vi "niRFUtil MEAS Peak Phase Correlation.vi"(2 "Pattern Signal":T1 {"y" format="%.2f"; "dx" format="%^.2e"; "x0" format="%^.2e"}, 3 "Signal In":T1 {"y" format="%.2f"; "dx" format="%^.2e"; "x0" format="%^.2e"}) -> (0 "Offset (s)":dbl format="%^.2e", 1 "Correlation Peak":sgl format="%^.2e")   [LabVIEW 2015, in "niRFUtil.lvlib"]
doc: "(c) Copyright 2006, National Instruments, Inc. This VI may not be duplicated, sold, or distributed without written consent from National Instruments."
uses:
  niRFUtil.lvlib
  Includes/niRFUtil INC Complex Waveform.ctl
  Includes/niRFUtil INC Complex Array.ctl
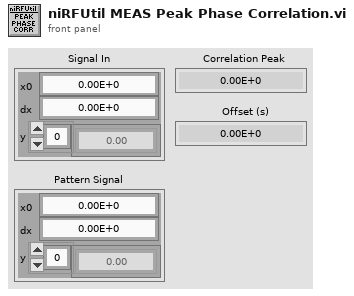
[diagram p1: front panel]
types:
  T1 = typedef "niRFUtil.lvlib/niRFUtil INC Complex Waveform.ctl" = cluster{"x0":dbl, "dx":dbl, "y":T2}
  T2 = typedef "niRFUtil.lvlib/niRFUtil INC Complex Array.ctl" = csg[]
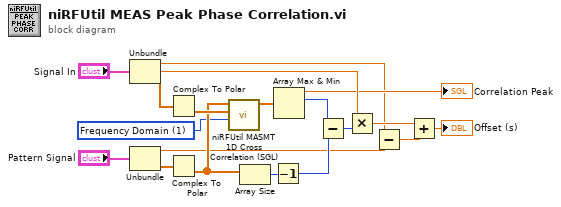
[diagram p0: block diagram]
diagram:
  w1 = 1 items=["Direct", "Frequency Domain"] ("algorithm")
  n1 = Unbundle("Signal In") -> ("x0"=w6:dbl, "dx"=w17:dbl, "y"=w3:T2)
  n2 = Unbundle("Pattern Signal") -> ("x0"=w5:dbl, "y"=w11:T2)  [unwired: 1 out]
  n3 = Complex To Polar(r * e^(i*theta)=w3) -> (theta=w19:sgl[])  [unwired: 1 out]
  n4 = Complex To Polar(r * e^(i*theta)=w11) -> (theta=w14:sgl[])  [unwired: 1 out]
  n5 = call "niRFUtil MASMT 1D Cross Correlation (SGL).vi"("algorithm"=w1, "Y"=w19, "X"=w14) -> ("Rxy"=w18:sgl[])  [unwired: 7 in, 1 out]
  n6 = Array Size(array=w14) -> (size(s)=w13:i32)
  n7 = Decrement(x=w13) -> (x-1=w12:i32)
  n8 = Array Max & Min(array=w18) -> (max value=→"Correlation Peak":sgl, max index (indices)=w16:i32)  [unwired: 2 out]
  n9 = Subtract(x=w16, y=w12) -> (x-y=w15:i32)
  n10 = Multiply(x=w17, y=w15) -> (x*y=w9:dbl)
  n11 = Subtract(x=w6, y=w5) -> (x-y=w4:dbl)
  n12 = Add(x=w9, y=w4) -> (x+y=→"Offset (s)":dbl)
